vi "INVERNADERO.vi"() -> ()   [LabVIEW 2018]
doc: "This example illustrates how to use a fuzzy controller to control a greenhouse system."
uses:
  <vilib>/addons/Fuzzy Logic/TypeDefs/FL System.ctl
  <vilib>/addons/Fuzzy Logic/TypeDefs/FL Variable.ctl
  <vilib>/addons/Fuzzy Logic/TypeDefs/FL Membership Function.ctl
  <vilib>/addons/Fuzzy Logic/TypeDefs/FL Membership Function Shape.ctl
  <vilib>/addons/Fuzzy Logic/TypeDefs/FL Rule.ctl
  <vilib>/addons/Fuzzy Logic/TypeDefs/FL Antecedent.ctl
  <vilib>/addons/Fuzzy Logic/TypeDefs/FL Modifier.ctl
  <vilib>/addons/Fuzzy Logic/TypeDefs/FL Antecedent Connective.ctl
  <vilib>/addons/Fuzzy Logic/TypeDefs/FL Consequent.ctl
  <vilib>/addons/Fuzzy Logic/TypeDefs/FL Consequent Implication.ctl
  <vilib>/addons/Fuzzy Logic/TypeDefs/FL Defuzzification.ctl
  <vilib>/addons/Fuzzy Logic/TypeDefs/FL Interpolating polynomials.ctl
  <vilib>/addons/Fuzzy Logic/TypeDefs/FL Input_Output.ctl
  <vilib>/MakerHub/LINX/Public/Peripherals/Analog/Analog Read 1 Chan.vi
  <vilib>/MakerHub/LINX/Public/Peripherals/PWM/PWM Set Duty Cycle 1 Chan.vi
  <vilib>/MakerHub/LINX/Public/Peripherals/Analog/Analog Read N Chans.vi
  <vilib>/MakerHub/LINX/Private/Local IO/LinxAnalogRead.vi
  <vilib>/MakerHub/LINX/Public/Utilities/Check Channel.vi
  <vilib>/MakerHub/LINX/Public/Utilities/Open Serial.vi
  <vilib>/MakerHub/LINX/Private/Utilties/Generate Error.vi
  <vilib>/addons/Fuzzy Logic/FL Fuzzy Controller (MIMO).vi
  <vilib>/MakerHub/LINX/Public/Peripherals/PWM/PWM Set Duty Cycle N Chans.vi
  <vilib>/addons/Fuzzy Logic/Membership/FL Get Membership Function (Fuzzy System).vi
  <vilib>/addons/Fuzzy Logic/Membership/FL Set Membership Function (Fuzzy System).vi
  <vilib>/addons/Fuzzy Logic/NI_Fuzzy_Logic_API.lvlib
  <vilib>/MakerHub/LINX/LMH-LINX.lvlib
panel:
  out "fuzzy system out":T1={"input variables"=[{"name"="Temperature", "range"=[0.0, 50.0, 0.0, 50.0], "MFs"=[{"name"="Cold", "shape"=1, "points"=[0.0, 0.0, 13.0, 21.0], "color"=42751, "user-defined shape index"=0}, {"name"="Normal", "shape"=3, "points"=[15.0, 20.0, 25.0, 30.0], "color"=16757760, "user-defined shape index"=0}, {"name"="Warm", "shape"=1, "points"=[24.0, 32.0, 50.0, 50.0], "color"=16714752, "user-defined shape index"=0}]}, {"name"="Humidity", "range"=[0.0, 100.0, 0.0, 100.0], "MFs"=[{"name"="Dry", "shape"=4, "points"=[0.0, 0.0, 10.0, 70.0], "color"=11796480, "user-defined shape index"=0}, {"name"="Normal", "shape"=4, "points"=[15.0, 68.0, 75.0, 90.0], "color"=16759338, "user-defined shape index"=0}, {"name"="Wet", "shape"=3, "points"=[70.0, 90.0, 100.0, 100.0], "color"=11861920, "user-defined shape index"=0}]}], "output variables"=[{"name"="Electric Roof", "range"=[0.0, 10.0, 0.0, 10.0], "MFs"=[{"name"="Closed", "shape"=0, "points"=[0.0, 0.0, 5.0], "color"=16711680, "user-defined shape index"=0}, {"name"="Semi-open", "shape"=0, "points"=[0.0, 5.0, 10.0], "color"=16774656, "user-defined shape index"=0}, {"name"="Open", "shape"=0, "points"=[5.0, 10.0, 10.0], "color"=2410496, "user-defined shape index"=0}]}, {"name"="Water Spills", "range"=[0.0, 10.0, 0.0, 10.0], "MFs"=[{"name"="Less", "shape"=0, "points"=[0.0, 0.0, 5.0], "color"=15263, "user-defined shape index"=0}, {"name"="Moderate", "shape"=0, "points"=[0.0, 5.0, 10.0], "color"=34559, "user-defined shape index"=0}, {"name"="More", "shape"=0, "points"=[5.0, 10.0, 10.0], "color"=2811647, "user-defined shape index"=0}]}], "rules"=[{"antecedents"=[{"Var Index"=0, "MF Index"=0, "Cond"=0}, {"Var Index"=1, "MF Index"=0, "Cond"=0}], "antecedent connective"=0, "consequents"=[{"Var Index"=0, "MF Index"=0, "Cond"=0}, {"Var Index"=1, "MF Index"=1, "Cond"=0}], "consequent implication"=1, "degree of support"=1.0}, {"antecedents"=[{"Var Index"=0, "MF Index"=0, "Cond"=0}, {"Var Index"=1, "MF Index"=1, "Cond"=0}], "antecedent connective"=0, "consequents"=[{"Var Index"=0, "MF Index"=0, "Cond"=0}, {"Var Index"=1, "MF Index"=0, "Cond"=0}], "consequent implication"=1, "degree of support"=1.0}, {"antecedents"=[{"Var Index"=0, "MF Index"=0, "Cond"=0}, {"Var Index"=1, "MF Index"=2, "Cond"=0}], "antecedent connective"=0, "consequents"=[{"Var Index"=0, "MF Index"=0, "Cond"=0}, {"Var Index"=1, "MF Index"=0, "Cond"=0}], "consequent implication"=1, "degree of support"=1.0}, {"antecedents"=[{"Var Index"=0, "MF Index"=1, "Cond"=0}, {"Var Index"=1, "MF Index"=0, "Cond"=0}], "antecedent connective"=0, "consequents"=[{"Var Index"=0, "MF Index"=1, "Cond"=0}, {"Var Index"=1, "MF Index"=2, "Cond"=0}], "consequent implication"=1, "degree of support"=1.0}, {"antecedents"=[{"Var Index"=0, "MF Index"=1, "Cond"=0}, {"Var Index"=1, "MF Index"=1, "Cond"=0}], "antecedent connective"=0, "consequents"=[{"Var Index"=0, "MF Index"=1, "Cond"=0}, {"Var Index"=1, "MF Index"=1, "Cond"=0}], "consequent implication"=1, "degree of support"=1.0}, {"antecedents"=[{"Var Index"=0, "MF Index"=1, "Cond"=0}, {"Var Index"=1, "MF Index"=2, "Cond"=0}], "antecedent connective"=0, "consequents"=[{"Var Index"=0, "MF Index"=1, "Cond"=0}, {"Var Index"=1, "MF Index"=0, "Cond"=0}], "consequent implication"=1, "degree of support"=1.0}, {"antecedents"=[{"Var Index"=0, "MF Index"=2, "Cond"=0}, {"Var Index"=1, "MF Index"=0, "Cond"=0}], "antecedent connective"=0, "consequents"=[{"Var Index"=0, "MF Index"=2, "Cond"=0}, {"Var Index"=1, "MF Index"=2, "Cond"=0}], "consequent implication"=1, "degree of support"=1.0}, {"antecedents"=[{"Var Index"=0, "MF Index"=2, "Cond"=0}, {"Var Index"=1, "MF Index"=1, "Cond"=0}], "antecedent connective"=0, "consequents"=[{"Var Index"=0, "MF Index"=2, "Cond"=0}, {"Var Index"=1, "MF Index"=1, "Cond"=0}], "consequent implication"=1, "degree of support"=1.0}, {"antecedents"=[{"Var Index"=0, "MF Index"=2, "Cond"=0}, {"Var Index"=1, "MF Index"=2, "Cond"=0}], "antecedent connective"=0, "consequents"=[{"Var Index"=0, "MF Index"=2, "Cond"=0}, {"Var Index"=1, "MF Index"=1, "Cond"=0}], "consequent implication"=1, "degree of support"=1.0}], "defuzzification method"=3, "description"="", "user MF interpolating polynomials"=[]} {"user MF interpolating polynomials"."coa_x(y) coeff" format="%.4g"; "user MF interpolating polynomials"."Area(y) coeff" format="%.4g"; "user MF interpolating polynomials"."X(y) coeff" format="%.4g"; "user MF interpolating polynomials"."Y(x) coeff" format="%.4g"; "user MF interpolating polynomials"."Y" format="%.4g"; "user MF interpolating polynomials"."X" format="%.4g"; "defuzzification method" items=["Center of Area", "Modified Center of Area", "Center of Sums", "Center of Maximum", "Mean of Maximum"]; "rules"."consequents"."Var Index" min=0; "rules"."consequents"."Cond" items=["=", "!="]; "rules"."consequents"."MF Index" min=0; "rules"."antecedents"."Var Index" min=0; "rules"."antecedents"."Cond" items=["=", "!="]; "rules"."antecedents"."MF Index" min=0; "rules"."consequent implication" items=["Minimum", "Product"]; "rules"."antecedent connective" items=["AND (Minimum)", "AND (Product)", "OR (Maximum)", "OR (Probabilistic)"]; "output variables"."MFs"."shape" items=["Triangle", "Trapezoid", "Singleton", "Sigmoid", "Gaussian", "User-Defined"]; "input variables"."MFs"."shape" items=["Triangle", "Trapezoid", "Singleton", "Sigmoid", "Gaussian", "User-Defined"]}
  in  "Tab Control":enum32{"", "Fuzzy Logic Invernadero"}(tab)
  out "Humedad (%)":dbl(slide) scale=0.0..100.0
  out "Temperatura (°C)":dbl(slide) scale=0.0..50.0
  in  "Season":dbl(knob) scale=5.0..-10.0
  out "%":dbl
  out "°C":dbl
  in  "Serial Port":refnum<visa-resource-name>="N/A"
  out "Membership functions for temperature":cluster{cluster{"Xi":dbl, "Yi":dbl}[]}[](graph)
  out "Intensidad de la Bomba":dbl(slide)=5.555555555555555 scale=0.0..10.0
  out "Intensidad del Ventilador":dbl(slide)=4.976391598507772 scale=0.0..10.0
  in  "Stop":bool
  # "IF"
  # "THEN"
  # "Invernadero \nUniversidad Politecnica de Aguascalientes\nMTR09D\nAlumnos:\nAlondra María Rodríguez Vázquez\nIsaías Gonzales Juárez\nMarco Antonio Mendoza Díaz\nRené Ulises Argüelles Gutiérrez"
  # "Spring"
  # "Fall"
  # "Summer"
  # "Winter"
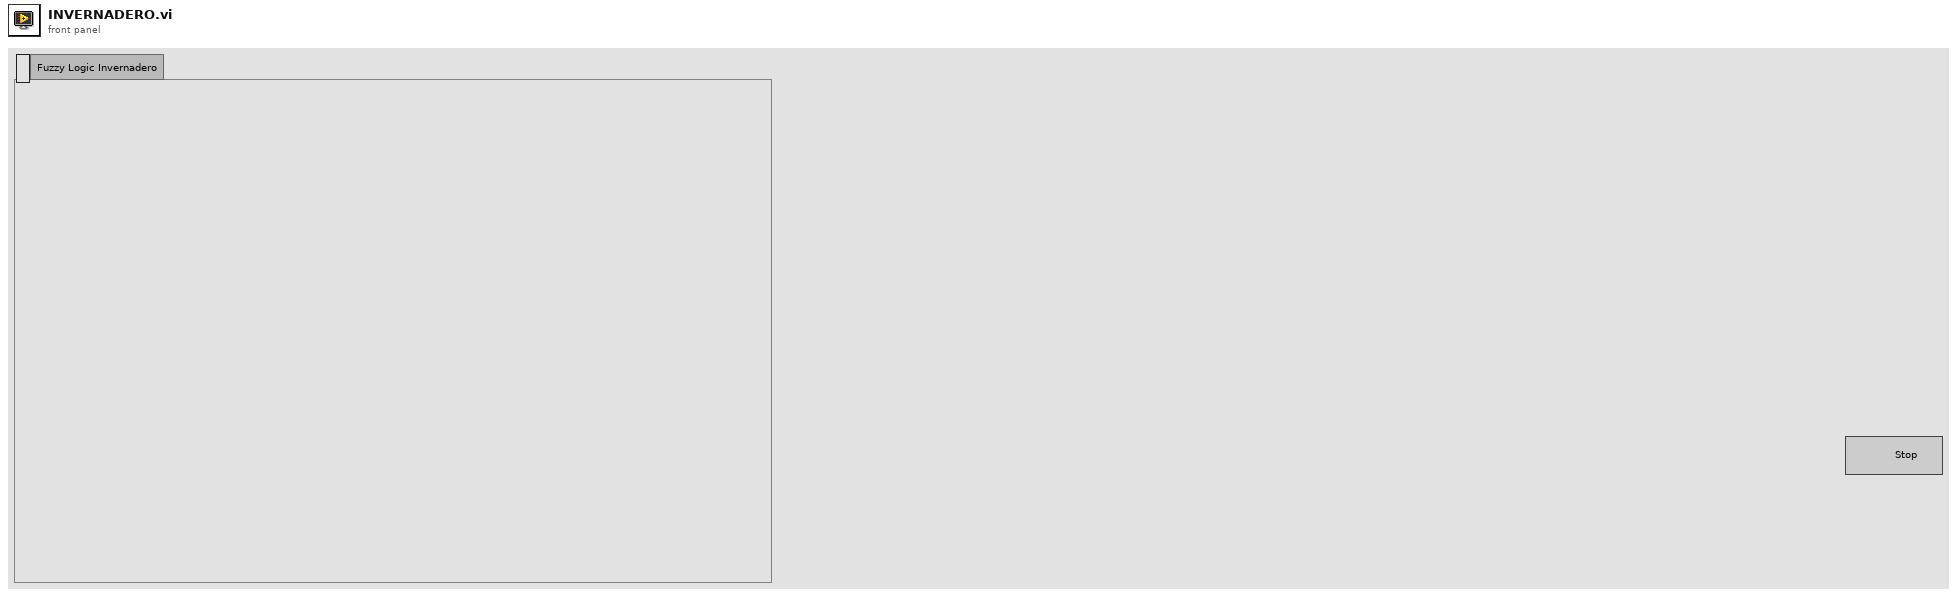
[diagram p1: front panel]
types:
  T1 = typedef "NI_Fuzzy_Logic_API.lvlib/FL System.ctl" = cluster{"input variables":T2[], "output variables":T2[], "rules":T5[], "defuzzification method":T11, "description":string, "user MF interpolating polynomials":T12[]}
  T2 = typedef "NI_Fuzzy_Logic_API.lvlib/FL Variable.ctl" = cluster{"name":string, "range":dbl[], "MFs":T3[]}
  T3 = typedef "NI_Fuzzy_Logic_API.lvlib/FL Membership Function.ctl" = cluster{"name":string, "shape":T4, "points":dbl[], "color":u32, "user-defined shape index":i32}
  T4 = typedef "NI_Fuzzy_Logic_API.lvlib/FL Membership Function Shape.ctl" = u16
  T5 = typedef "NI_Fuzzy_Logic_API.lvlib/FL Rule.ctl" = cluster{"antecedents":T6[], "antecedent connective":T8, "consequents":T9[], "consequent implication":T10, "degree of support":dbl}
  T6 = typedef "NI_Fuzzy_Logic_API.lvlib/FL Antecedent.ctl" = cluster{"Var Index":i32, "MF Index":i32, "Cond":T7}
  T7 = typedef "NI_Fuzzy_Logic_API.lvlib/FL Modifier.ctl" = u16
  T8 = typedef "NI_Fuzzy_Logic_API.lvlib/FL Antecedent Connective.ctl" = u16
  T9 = typedef "NI_Fuzzy_Logic_API.lvlib/FL Consequent.ctl" = cluster{"Var Index":i32, "MF Index":i32, "Cond":T7}
  T10 = typedef "NI_Fuzzy_Logic_API.lvlib/FL Consequent Implication.ctl" = u16
  T11 = typedef "NI_Fuzzy_Logic_API.lvlib/FL Defuzzification.ctl" = u16
  T12 = typedef "NI_Fuzzy_Logic_API.lvlib/FL Interpolating polynomials.ctl" = cluster{"X":dbl[], "Y":dbl[], "Y(x) coeff":dbl[][], "X(y) coeff":dbl[][], "Area(y) coeff":dbl[][], "coa_x(y) coeff":dbl[][]}
  T13 = typedef "LMH-LINX.lvlib/LINX Ref.ctl" = cluster{"IO":T14, "Interface":T15, "LINX Device Config":T16}
  T14 = typedef "LMH-LINX.lvlib/Platform.ctl" = enum16{"Remote", "Local"}
  T15 = typedef "LMH-LINX.lvlib/Interface.ctl" = enum16{"Serial", "TCP"}
  T16 = typedef "LMH-LINX.lvlib/Device.lvlib/LINX Device Config.ctl" = cluster{"Interface":T15, "COM Port":refnum<visa-resource-name>, "TCP Configuration":T17, "Device Family":u8, "Device ID":u8, "Device Name":string, "TCP Ref":refnum<k5>, "Channels":T18}
  T17 = typedef "LMH-LINX.lvlib/Device.lvlib/TCP Config.ctl" = cluster{"IP Address":string, "Port":u16}
  T18 = typedef "LMH-LINX.lvlib/Channels.ctl" = cluster{"DI":u8[], "DO":u8[], "AI":u8[], "AO":u8[], "PWM":u8[], "QE":u8[], "UART":u8[], "I2C 2":u8[], "SPI":u8[], "CAN":u8[], "Servo":u8[], "AI Ref (V)":dbl, "AI Resolution (Bits)":u8, "AO Ref (V)":dbl, "AO Resolution (Bits)":u8}
  T19 = typedef "NI_Fuzzy_Logic_API.lvlib/FL Input_Output.ctl" = u16
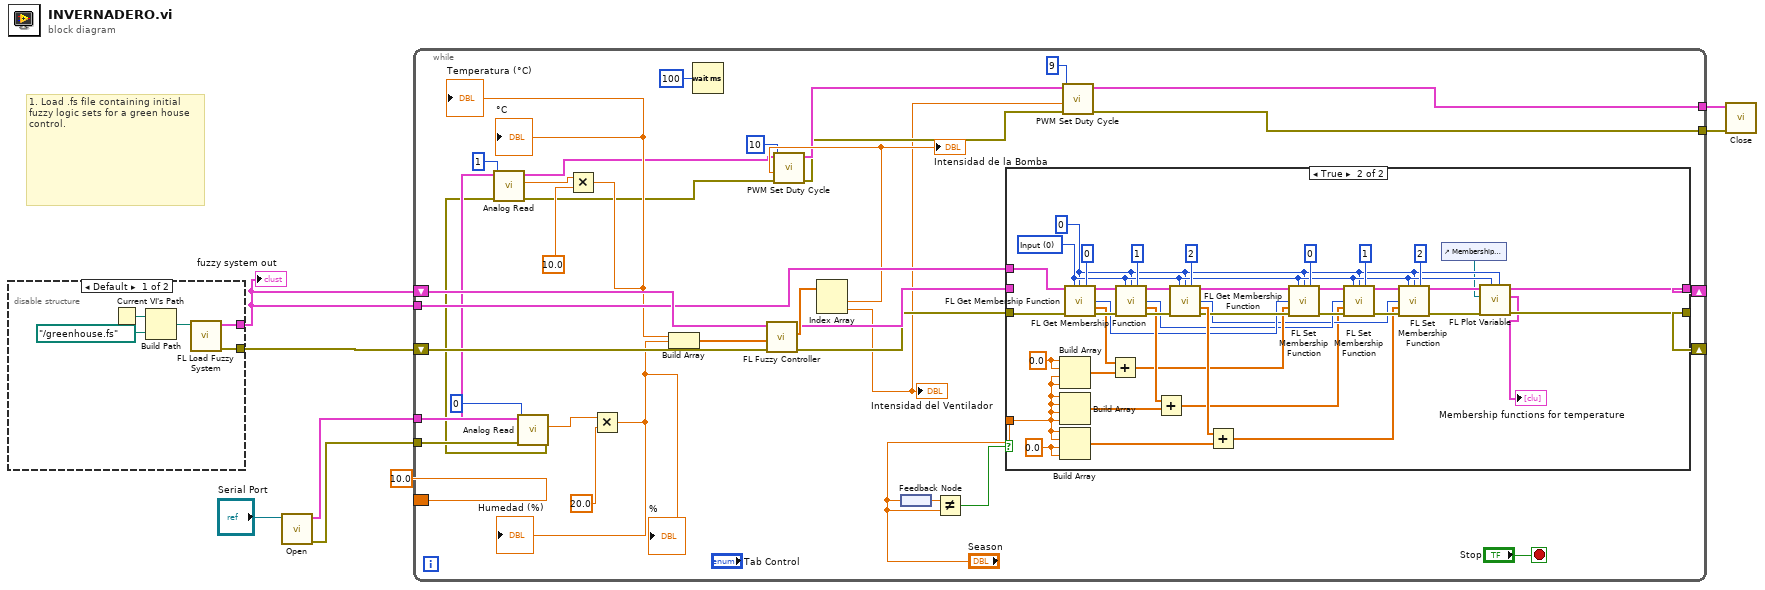
[diagram p0: block diagram]
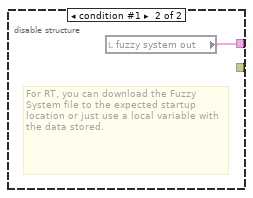
[diagram p2: hidden frame]
diagram:
  # "1. Load .fs file containing initial fuzzy logic sets for a green house control."
  n1 = disable-structure shown="Default" {
    disable-tunnel: [w13 _] -> w8
    disable-tunnel: [w12 w14] -> w7
    frame condition #0 (active) {
      n2 = Current VI's Path() -> (path=w11:path)
      n3 = Build Path(base path=w11, name or relative path=path "../greenhouse.fs") -> (appended path=w9:path)
      n4 = call <vilib>:"FL Load Fuzzy System.vi"("file path"=w9) -> ("error out"=w13:errorcluster, "fuzzy system out"=w12:T1)  [unwired: 1 in, 8 out]
    }
    frame condition #1 {
      # "For RT, you can download the Fuzzy System file to the expected startup location or just use a local variable with the data stored."
      n5 = local read "fuzzy system out"() -> (w14:T1)
    }
  }
  "fuzzy system out" <- w7
  n6 = call-poly <vilib>:"Open.vi"("Serial Port"="Serial Port") -> ("Error Out"=w3:errorcluster, "LINX Resource"=w4:T13)  [unwired: 8 in, 1 out]
  n7 = while {
    shift-right: [w41] -> _
    shift-left: w7 -> [w39]
    shift-right: [w42] -> _
    shift-left: w8 -> [w49]
    tunnel: w7 -> [w38]
    border: 10.0 ("Season") -> [_]
    tunnel: w4 -> [w36]
    tunnel: w3 -> [w35]
    tunnel: [w21] -> w2
    tunnel: [w20] -> w1
    stop <- "Stop" stop-if-true
    n8 = call-poly <vilib>:"Analog Read.vi"("Error In"=w35, "Analog Channel"=u8 0, "LINX Resource"=w36) -> ("Error Out"=w29:errorcluster, "Voltage"=w19:dbl, "LINX Resource"=w30:T13)  [unwired: 5 in, 1 out]
    n9 = call-poly <vilib>:"Analog Read.vi"("Error In"=w29, "Analog Channel"=u8 1, "LINX Resource"=w30) -> ("Error Out"=w15:errorcluster, "Voltage"=w33:dbl, "LINX Resource"=w16:T13)  [unwired: 5 in, 1 out]
    n10 = Multiply(x=w33, y=10.0) -> (x*y=w31:dbl)
    "°C" <- w31
    "Temperatura (°C)" <- w31
    n11 = Multiply(x=w19, y=20.0) -> (x*y=w17:dbl)
    "%" <- w17
    "Humedad (%)" <- w17
    n12 = Build Array(w31, w17) -> (w37:dbl[])
    n13 = Wait (ms)(milliseconds to wait=u32 100) -> ()  [unwired: 1 out]
    n14 = call-poly <vilib>:"FL Fuzzy Controller.vi"("error in (no error)"=w49, "input values"=w37, "fuzzy system in"=w39) -> ("error out"=w43:errorcluster, "output values"=w48:dbl[], "fuzzy system out"=w44:T1)  [unwired: 6 out]
    n15 = Index Array(array=w48) -> (element #1=w27:dbl, element #2=w23:dbl)  [unwired: 2 in]
    "Intensidad de la Bomba" <- w27
    "Intensidad del Ventilador" <- w23
    n16 = call-poly <vilib>:"PWM Set Duty Cycle.vi"("Error In"=w15, "Duty Cycle (0-1)"=w27, "PWM Channel"=u8 10, "LINX Resource"=w16) -> ("Error Out"=w24:errorcluster, "LINX Resource"=w25:T13)  [unwired: 6 in]
    n17 = feedback-in #1("Season") -> ()
    n18 = feedback #1() -> (w46:dbl)
    n19 = Not Equal?(x=w46, y="Season") -> (x != y?=w45:bool)
    n20 = case shown="True" w45 {
      tunnel: w44 -> [w52 _]
      tunnel: w43 -> [w51 w93]
      tunnel: [w51 w57] -> w42
      tunnel: [w52 w59] -> w41
      tunnel: "Season" -> [_ w87]
      tunnel: w38 -> [_ w92]
      frame False {
        # "Does not change controller parameters if not needed"
      }
      frame True {
        w66 = 0.0 ("element")
        w68 = 0.0 ("element")
        w55 = 0 ("Var index")
        w56 = T19 0 items=["Input", "Output"] ("Input/Output")
        n21 = Build Array(w68, w68, w87, w87) -> (w85:dbl[])
        n22 = Build Array(w87, w87, w87, w87) -> (w84:dbl[])
        n23 = Build Array(w87, w87, w66, w66) -> (w82:dbl[])
        n24 = call-poly <vilib>:"FL Get Membership Function.vi"("fuzzy system in"=w92, "input/output"=w56, "variable index"=w55, "membership function index"=0 ("MF index"), "error in (no error)"=w93) -> ("fuzzy system out"=w91:T1, "shape"=w71:T4, "points"=w86:dbl[], "error out"=w90:errorcluster)  [unwired: 7 out]
        n25 = Add(x=w86, y=w85) -> (x+y=w73:dbl[])
        n26 = call-poly <vilib>:"FL Get Membership Function.vi"("fuzzy system in"=w91, "input/output"=w56, "variable index"=w55, "membership function index"=1 ("MF index"), "error in (no error)"=w90) -> ("fuzzy system out"=w89:T1, "shape"=w70:T4, "points"=w83:dbl[], "error out"=w88:errorcluster)  [unwired: 7 out]
        n27 = Add(x=w83, y=w84) -> (x+y=w67:dbl[])
        n28 = call-poly <vilib>:"FL Get Membership Function.vi"("fuzzy system in"=w89, "input/output"=w56, "variable index"=w55, "membership function index"=2 ("MF index"), "error in (no error)"=w88) -> ("fuzzy system out"=w80:T1, "shape"=w69:T4, "points"=w81:dbl[], "error out"=w79:errorcluster)  [unwired: 7 out]
        n29 = Add(x=w81, y=w82) -> (x+y=w72:dbl[])
        n30 = call-poly <vilib>:"FL Set Membership Function.vi"("fuzzy system in"=w80, "input/output"=w56, "variable index"=w55, "membership function index"=0 ("MF index"), "shape"=w71, "points"=w73, "error in (no error)"=w79) -> ("fuzzy system out"=w76:T1, "error out"=w75:errorcluster)  [unwired: 3 in, 4 out]
        n31 = call-poly <vilib>:"FL Set Membership Function.vi"("fuzzy system in"=w76, "input/output"=w56, "variable index"=w55, "membership function index"=1 ("MF index"), "shape"=w70, "points"=w67, "error in (no error)"=w75) -> ("fuzzy system out"=w78:T1, "error out"=w77:errorcluster)  [unwired: 3 in, 4 out]
        n32 = call-poly <vilib>:"FL Set Membership Function.vi"("fuzzy system in"=w78, "input/output"=w56, "variable index"=w55, "membership function index"=2 ("MF index"), "shape"=w69, "points"=w72, "error in (no error)"=w77) -> ("fuzzy system out"=w60:T1, "error out"=w58:errorcluster)  [unwired: 3 in, 4 out]
        n33 = control-ref of="Membership functions for temperature"() -> (w54:refnum<vi>)
        n34 = call <vilib>:"FL Plot Variable.vi"("variable index"=w55, "input/output"=w56, "error in (no error)"=w58, "graph refnum"=w54, "fuzzy system in"=w60) -> ("error out"=w57:errorcluster, "membership functions plot"=→"Membership functions for temperature":cluster{cluster{"Xi":dbl, "Yi":dbl}[]}[], "fuzzy system out"=w59:T1)  [unwired: 4 out]
      }
    }
    n35 = call-poly <vilib>:"PWM Set Duty Cycle.vi"("Error In"=w24, "Duty Cycle (0-1)"=w23, "PWM Channel"=u8 9, "LINX Resource"=w25) -> ("Error Out"=w20:errorcluster, "LINX Resource"=w21:T13)  [unwired: 6 in]
  }
  n36 = call <vilib>:"Close.vi"("Error In"=w1, "LINX Resource"=w2) -> ()  [unwired: 9 in, 1 out]
